vi "getXMLArray.vi"(9 "size":i32, 11 "Array Node":refnum<k20>) -> (3 "Array":cluster{dbl, dbl}[](graph))   [LabVIEW 2013]
uses:
  <vilib>/xml/NI_XML.lvlib
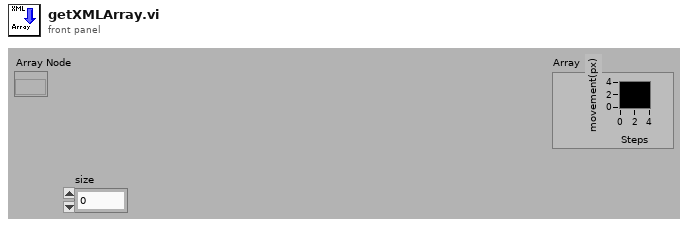
[diagram p1: front panel]
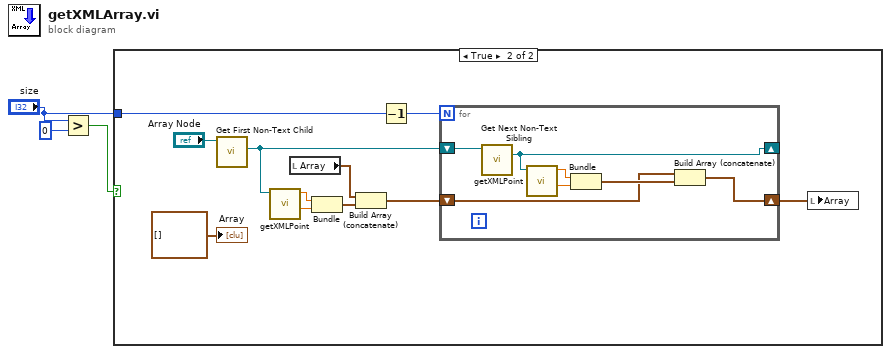
[diagram p0: block diagram]
diagram:
  n1 = Greater?(x="size", y=0) -> (0:w1:bool)
  n2 = case shown="True" w1 {
    tunnel: "size" -> [_ w4]
    frame False {
    }
    frame True {
      n3 = call <vilib>:"Get First Non-Text Child.vi"("node in"="Array Node") -> ("child node"=w7:refnum<k20>)  [unwired: 7 in, 3 out]
      n4 = call "getXMLPoint.vi"("Point Node"=w7) -> ("y"=w10:dbl, "x"=w11:dbl)  [unwired: 9 in]
      n5 = local read "Array"() -> (w8:cluster{dbl, dbl}[])
      n6 = Bundle("x"=w11, "y"=w10) -> (w12:cluster{"x":dbl, "y":dbl})  [unwired: 1 in]
      n7 = Build Array (concatenate)(w8, w12) -> (w6:cluster{"x":dbl, "y":dbl}[])
      n8 = Decrement(x=w4) -> (x-1=w13:i32)
      n9 = for {
        N: w13 -> [_]
        shift-right: [w17] -> _
        shift-left: w7 -> [w18]
        shift-right: [w16] -> w5
        shift-left: w6 -> [w15]
        n10 = call <vilib>:"Get Next Non-Text Sibling.vi"("node in"=w18) -> ("sibling node"=w17:refnum<k20>)  [unwired: 7 in, 3 out]
        n11 = call "getXMLPoint.vi"("Point Node"=w17) -> ("y"=w21:dbl, "x"=w20:dbl)  [unwired: 9 in]
        n12 = Bundle("x"=w20, "y"=w21) -> (w19:cluster{"x":dbl, "y":dbl})  [unwired: 1 in]
        n13 = Build Array (concatenate)(w15, w19) -> (w16:cluster{"x":dbl, "y":dbl}[])
      }
      n14 = local write "Array"(w5) -> ()
      "Array" <- cluster{dbl, dbl}[] [] ("Array")
    }
  }
